vi "Interpret Header.vi"(5 "Header":string="HTTP/1.1 100 Continue\r\n\r\nHTTP/1.1 400 Bad Request\r\nDate: Wed, 28 Sep 2022 17:22:04 GMT\r\nContent-Type: application/json\r\nContent-Length: 342\r\nConnection: keep-alive\r\nServer: gunicorn\r\nVary: Accept, Cookie\r\nAllow: GET, PUT, PATCH, HEAD, OPTIONS\r\nX-Frame-Options: DENY\r\nX-Content-Type-Options: nosniff\r\nReferrer-Policy: same-origin\r\nCross-Origin-Opener-Policy: same-origin\r\n\r\n", 11 "error in (no error)":errorcluster) -> (4 "HTTP response code":T1, 6 "Header (dup)":string="HTTP/1.1 301 Moved Permanently\r\nLocation: http://www.google.com/\r\nContent-Type: text/html; charset=UTF-8\r\nDate: Thu, 22 Mar 2012 21:41:48 GMT\r\nExpires: Sat, 21 Apr 2012 21:41:48 GMT\r\nCache-Control: public, max-age=2592000\r\nServer: gws\r\nContent-Length: 219\r\nX-XSS-Protection: 1; mode=block\r\nX-Frame-Options: SAMEORIGIN", 10 "Header Values":T2[](array[typedef]), 15 "error out":errorcluster)   [LabVIEW 2020, in "Blue Easy HTTP OpenSource.lvlib"]
doc: "Parses HTTP Header into array of headers and corresponding values."
uses:
  Blue Easy HTTP OpenSource.lvlib
  HTTP Header.ctl
  HTTP response code.ctl
  <vilib>/Utility/error.llb/whitespace.ctl
panel:
  # "HTTP/1.1 301 Moved Permanently\nLocation: http://www.google.com/\nContent-Type: text/html; charset=UTF-8\nDate: Thu, 22 Mar 2012 21:41:48 GMT\nExpires: Sat, 21 Apr 2012 21:41:48 GMT\nCache-Control: public, max-age=2592000\nServer: gws\nContent-Length: 219\nX-XSS-Protection: 1; mode=block\nX-Frame-Options: SAMEORIGIN"
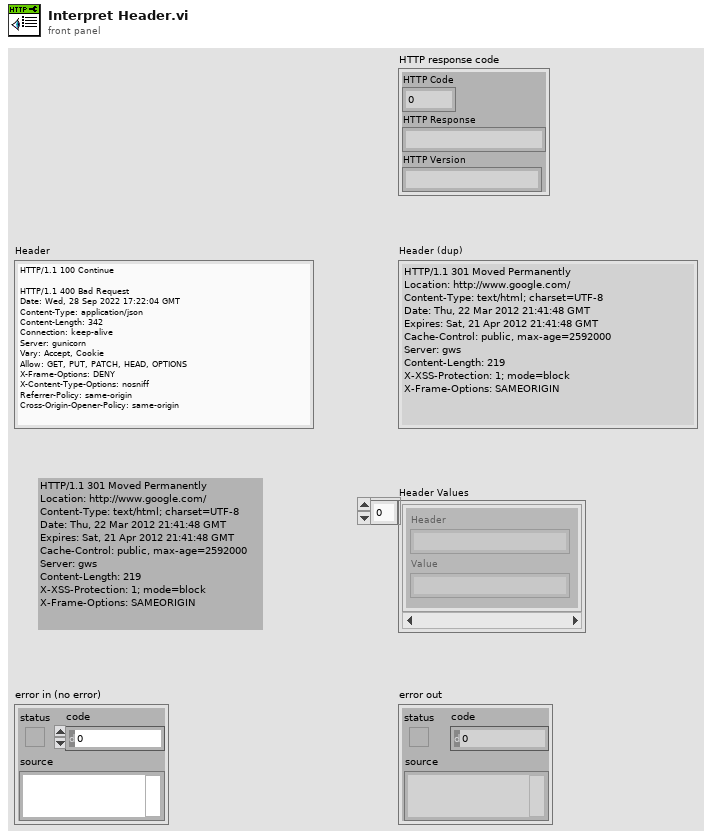
[diagram p1: front panel]
types:
  T1 = typedef "Blue Easy HTTP OpenSource.lvlib/HTTP response code.ctl" = cluster{"HTTP Code":u16, "HTTP Response":string, "HTTP Version":string}
  T2 = typedef "Blue Easy HTTP OpenSource.lvlib/HTTP Header.ctl" = cluster{"Header":string, "Value":string}
  T3 = typedef "whitespace.ctl" = u16
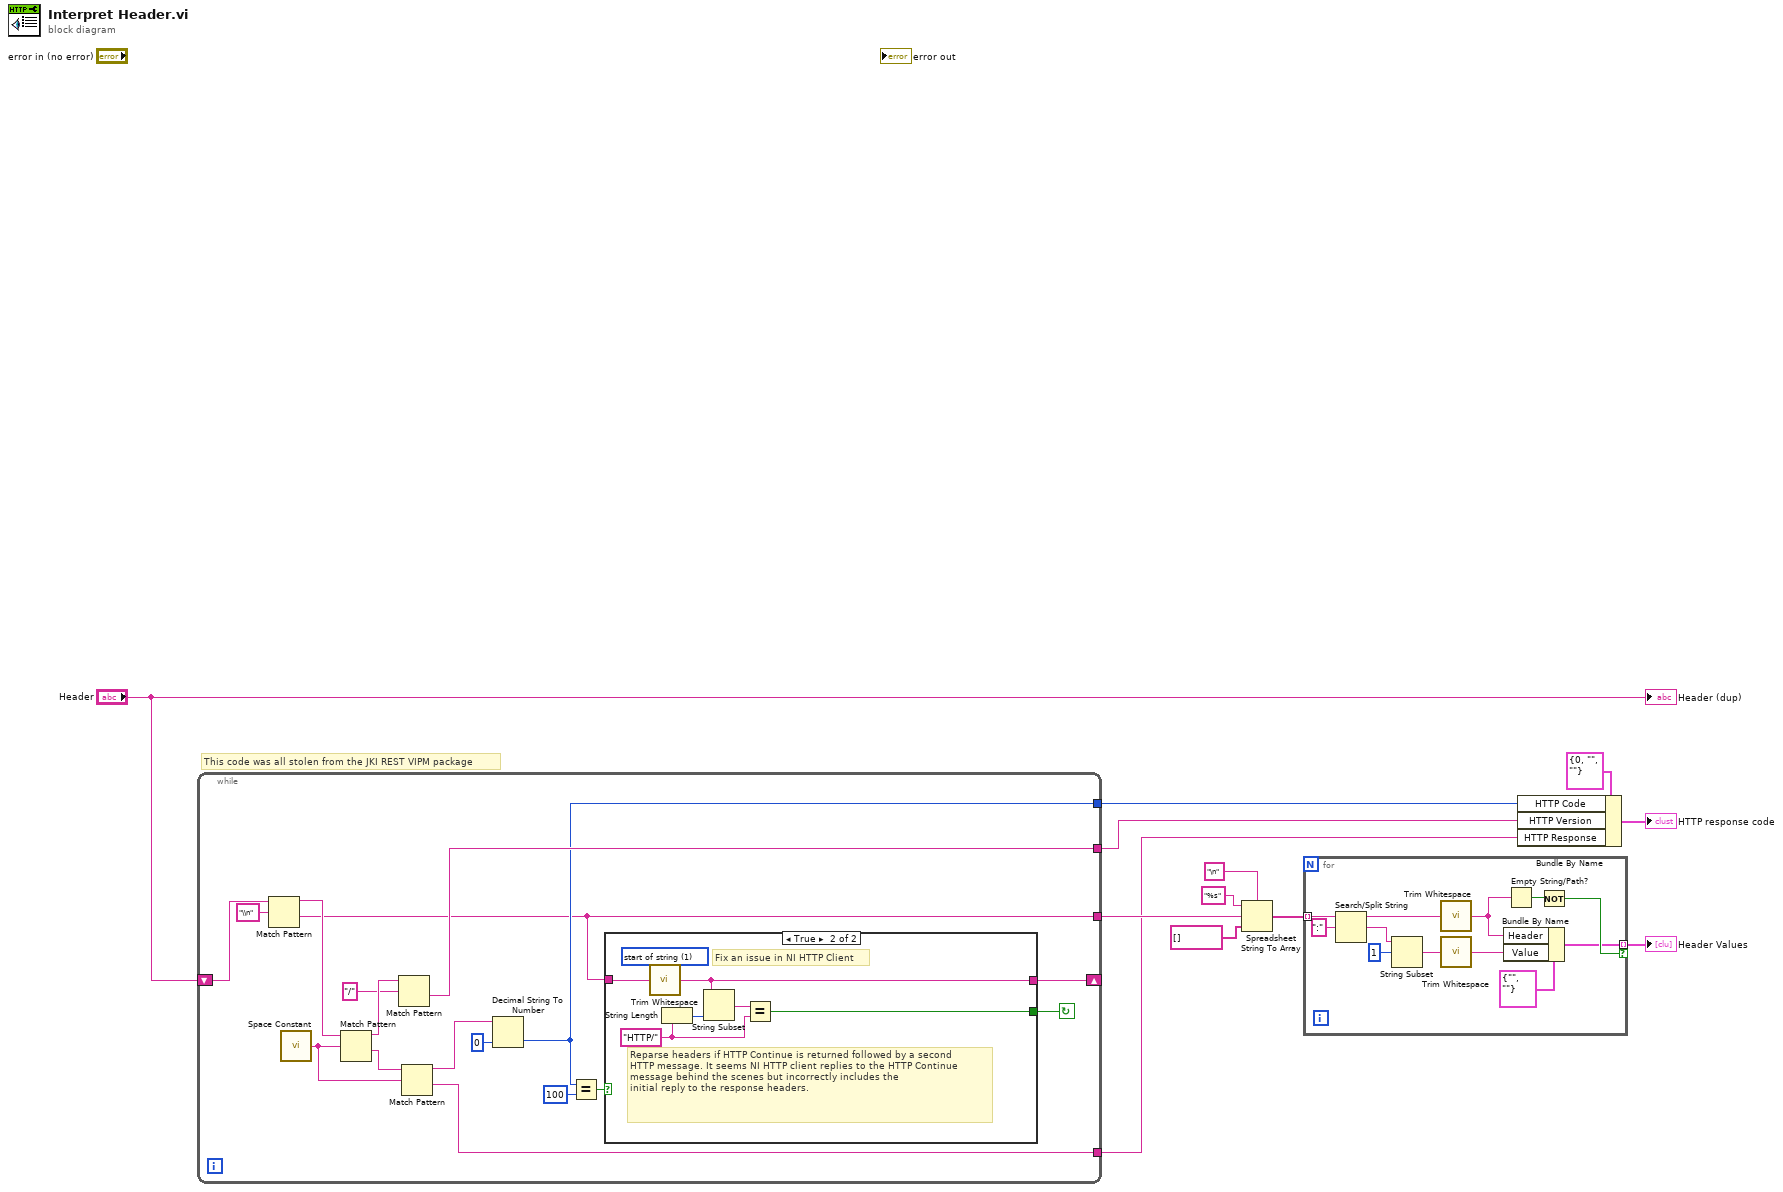
[diagram p0: block diagram]
diagram:
  # "This code was all stolen from the JKI REST VIPM package"
  n1 = while {
    shift-right: [w13] -> _
    shift-left: "Header" -> [w29]
    tunnel: [w15] -> w5
    tunnel: [w25] -> w2
    tunnel: [w18] -> w10
    tunnel: [w22] -> w1
    stop <- w14 continue-if-true
    n2 = Match Pattern(string=w29, regular expression="\\n") -> (before substring=w28:string, after substring=w15:string)  [unwired: 1 in, 2 out]
    n3 = call <vilib>:"Space Constant.vi"() -> ("String"=w23:string)
    n4 = Match Pattern(string=w28, regular expression=w23) -> (before substring=w27:string, after substring=w24:string)  [unwired: 1 in, 2 out]
    n5 = Match Pattern(string=w27, regular expression="/") -> (after substring=w25:string)  [unwired: 1 in, 3 out]
    n6 = Match Pattern(string=w24, regular expression=w23) -> (before substring=w20:string, after substring=w22:string)  [unwired: 1 in, 2 out]
    n7 = Decimal String To Number(string=w20, default (0L)=u16 0 ("default (0 I32)")) -> (number=w18:u16)  [unwired: 1 in, 1 out]
    n8 = Equal?(x=w18, y=u16 100) -> (x = y?=w16:bool)
    n9 = case shown="True" w16 {
      tunnel: w15 -> [_ w35]
      tunnel: [_ w31] -> w14
      tunnel: [_ w30] -> w13
      frame False {
      }
      frame True {
        w32 = "HTTP/"
        w36 = T3 1 items=["both", "start of string", "end of string"] ("location (both)")
        # "Fix an issue in NI HTTP Client"
        # "Reparse headers if HTTP Continue is returned followed by a second\nHTTP message. It seems NI HTTP client replies to the HTTP Continue message behind the scenes but incorrectly includes the\ninitial reply to the response headers."
        n10 = call <vilib>:"Trim Whitespace.vi"("string"=w35, "location (both)"=w36) -> ("trimmed string"=w30:string)
        n11 = String Length(string=w32) -> (length=w34:i32)
        n12 = String Subset(string=w30, length (rest)=w34) -> (substring=w33:string)  [unwired: 1 in]
        n13 = Equal?(x=w33, y=w32) -> (x = y?=w31:bool)
      }
    }
  }
  n14 = Spreadsheet String To Array(delimiter (Tab)="\n", format string="%s", spreadsheet string=w5, array type (2D Dbl)=string[] []) -> (array=w6:string[])
  n15 = for {
    tunnel: w6 -> [w48] mode=indexing
    tunnel: [w37] -> w3 mode=indexing if=w42
    n16 = Search/Split String(string=w48, search string/char (-)=":") -> (substring before match=w41:string, match + rest of string=w46:string)  [unwired: 1 in, 1 out]
    n17 = String Subset(string=w46, offset (0)=1) -> (substring=w44:string)  [unwired: 1 in]
    n18 = call <vilib>:"Trim Whitespace.vi"("string"=w41) -> ("trimmed string"=w38:string)  [unwired: 1 in]
    n19 = call <vilib>:"Trim Whitespace.vi"("string"=w44) -> ("trimmed string"=w39:string)  [unwired: 1 in]
    n20 = Bundle By Name(cluster=T2 {"Header"="", "Value"=""} ("HTTP Header"), "Header"=w38, "Value"=w39) -> (w37:T2)
    n21 = Empty String/Path?(string/path=w38) -> (empty?=w43:bool)
    n22 = Not(x=w43) -> (.not. x?=w42:bool)
  }
  "Header Values" <- w3
  n23 = Bundle By Name(cluster=T1 {"HTTP Code"=0, "HTTP Response"="", "HTTP Version"=""} ("Cluster"), "HTTP Code"=w10, "HTTP Version"=w2, "HTTP Response"=w1) -> (→"HTTP response code":T1)
  "Header (dup)" <- "Header"
